vi "Request_int_str.vi"(0 "reference in":T1, 5 "method":string, 7 "params":variant, 9 "id":i32, 11 "error in (no error)":errorcluster) -> (4 "reference out":T1, 6 "response":string, 15 "error out":errorcluster)   [LabVIEW 2017, in "JSON_RPC_client.lvlib"]
uses:
  JSON_RPC_client.lvlib
  reference.ctl
  <vilib>/httpClient/ClientHandle.ctl
  <vilib>/LVH/i3 JSON/JSON Generation/Create Value Files/Create Value - Object.vi
  <vilib>/LVH/i3 JSON/JSON Generation/Add Object Parameter Files/Add Object Parameter - String.vi
  <vilib>/LVH/i3 JSON/JSON Generation/Add Object Parameter Files/Add Object Parameter - Numeric.vi
  <vilib>/httpClient/POSTBuffer.vi
  <vilib>/httpClient/LabVIEWHTTPClient.lvlib
  <vilib>/LVH/i3 JSON/i3-json.lvlib
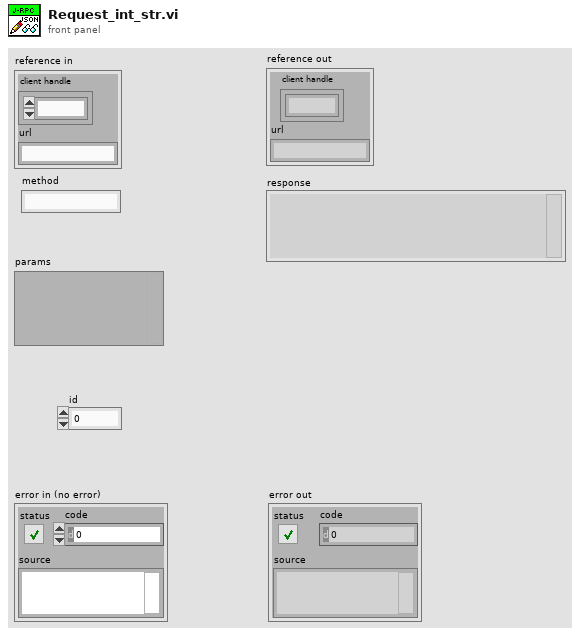
[diagram p1: front panel]
types:
  T1 = typedef "JSON_RPC_client.lvlib/reference.ctl" = cluster{"client handle":T2, "url":string}
  T2 = typedef "LabVIEWHTTPClient.lvlib/ClientHandle.ctl" = refnum<k1>
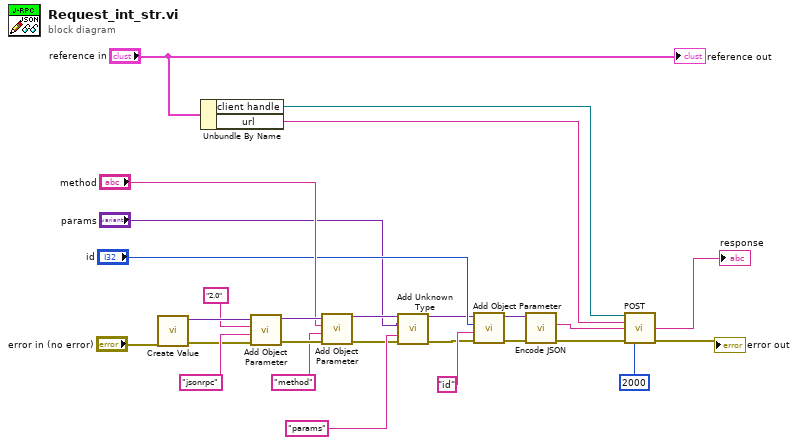
[diagram p0: block diagram]
diagram:
  n1 = call-poly <vilib>:"Create Value.vi"("error in (no error)"="error in (no error)") -> ("error out"=w18:errorcluster, "JSON Tree"=w22:variant)  [unwired: 9 in]
  n2 = Unbundle By Name("reference in") -> ("client handle"=w24:T2, "url"=w23:string)
  n3 = call-poly <vilib>:"Add Object Parameter.vi"("error in (no error)"=w18, "Name"="jsonrpc", "String"="2.0", "JSON Tree in (JSON Object)"=w22) -> ("error out"=w16:errorcluster, "JSON Tree out (JSON Object)"=w17:variant)  [unwired: 6 in]
  n4 = call-poly <vilib>:"Add Object Parameter.vi"("error in (no error)"=w16, "Name"="method", "String"="method", "JSON Tree in (JSON Object)"=w17) -> ("error out"=w2:errorcluster, "JSON Tree out (JSON Object)"=w6:variant)  [unwired: 6 in]
  n5 = call "Add Unknown Type.vi"("JSON Tree out (JSON Object) in"=w6, "result"="params", "Name"="params", "error in (no error)"=w2) -> ("JSON Tree out (JSON Object) out"=w5:variant, "error out"=w7:errorcluster)  [unwired: 10 in]
  n6 = call-poly <vilib>:"Add Object Parameter.vi"("error in (no error)"=w7, "Name"="id", "Numeric"="id", "JSON Tree in (JSON Object)"=w5) -> ("error out"=w11:errorcluster, "JSON Tree out (JSON Object)"=w10:variant)  [unwired: 6 in]
  n7 = call <vilib>:"Encode JSON.vi"("error in (no error)"=w11, "JSON Tree"=w10) -> ("error out"=w8:errorcluster, "String"=w9:string)  [unwired: 4 in]
  n8 = call-poly <vilib>:"POST.vi"("client handle"=w24, "url"=w23, "buffer"=w9, "error in (no error)"=w8, "timeout (10000)"=2000) -> ("body"=→"response":string, "error out"=→"error out":errorcluster)  [unwired: 7 in, 2 out]
  "reference out" <- "reference in"
